vi "DeleteFileFlowStep.vi"(8 "error in (no error)":errorcluster, 11 "Fileflow step":string) -> (0 "error out":errorcluster)   [LabVIEW 2017, in "FileFlow.lvlib"]
doc: "Removes a process from the Fileflow Script."
uses:
  <vilib>/addons/InsightCM/Devices/Shared/Common/FileFlow/FileFlow.lvlib
  <vilib>/addons/InsightCM/Devices/Shared/Common/DataFlow/DataFlow.lvlib
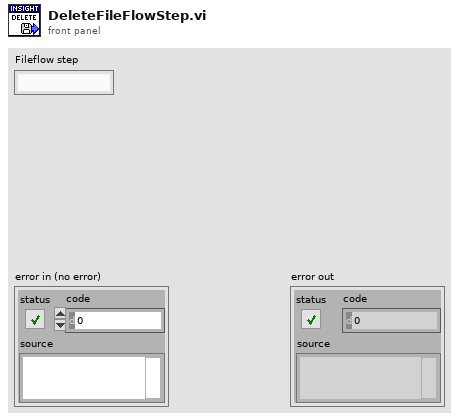
[diagram p1: front panel]
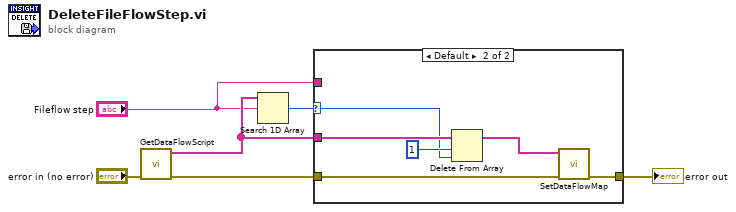
[diagram p0: block diagram]
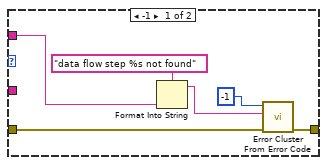
[diagram p2: hidden frame]
diagram:
  n1 = call <vilib>:"GetDataFlowScript.vi"("error in (no error)"="error in (no error)") -> ("error out"=w3:errorcluster, "Dataflow script"=w4:string[])  [unwired: 8 in, 1 out]
  n2 = Search 1D Array(1D array=w4, element="Fileflow step") -> (index of element=w5:i32)  [unwired: 1 in]
  n3 = case shown="Default" w5 {
    selector: w5 -> [_ w16]
    tunnel: w4 -> [_ w18]
    tunnel: w3 -> [w12 w15]
    tunnel: [w11 w14] -> w1
    tunnel: "Fileflow step" -> [w9 _]
    frame -1 {
      n4 = Format Into String(format string="data flow step %s not found", w9) -> (resulting string=w8:string)  [unwired: 2 in, 1 out]
      n5 = call <vilib>:"Error Cluster From Error Code.vi"("error in (no error)"=w12, "error message (\"\")"=w8, "error code (0)"=-1) -> ("error out"=w11:errorcluster)  [unwired: 6 in]
    }
    frame Default {
      n6 = Delete From Array(array=w18, length=1, index=w16) -> (array with subset deleted=w13:string[])  [unwired: 1 out]
      n7 = call <vilib>:"SetDataFlowMap.vi"("error in (no error)"=w15, "Dataflow script"=w13) -> ("error out"=w14:errorcluster)  [unwired: 9 in]
    }
  }
  "error out" <- w1
